vi "getCurrent.vi"(3 "error in (no error)":errorcluster, 4 "Throttle % [0-100]":dbl, 5 "Ammeter in":refnum<class "Ammeter.lvclass">) -> (0 "error out":errorcluster, 1 "Current [Amps]":dbl, 2 "Ammeter out":refnum<class "Ammeter.lvclass">)   [LabVIEW 2015, in "Ammeter.lvclass"]
uses:
  Ammeter.lvclass
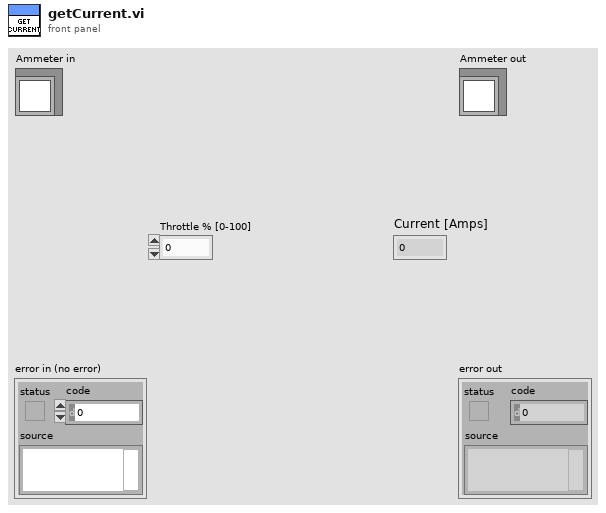
[diagram p1: front panel]
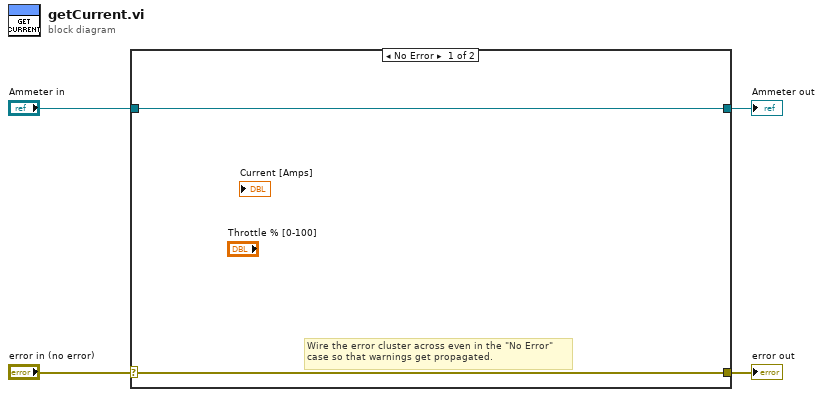
[diagram p0: block diagram]
diagram:
  n1 = case shown="No Error" "error in (no error)" {
    selector: "error in (no error)" -> [w5 w8]
    tunnel: [w5 w8] -> w3
    tunnel: [w6 w7] -> w1
    tunnel: "Ammeter in" -> [w6 w7]
    frame No Error {
      # "Wire the error cluster across even in the \"No Error\"\ncase so that warnings get propagated."
    }
    frame Error {
    }
  }
  "error out" <- w3
  "Ammeter out" <- w1
